vi "UART Clear Buffer.vi"(5 "Error In":errorcluster, 8 "VISA Resource In":refnum<visa-resource-name>="COM1") -> (0 "Error Out":errorcluster, 3 "VISA Resource Out":refnum<visa-resource-name>)   [LabVIEW 2015]
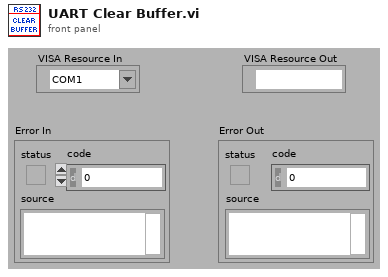
[diagram p1: front panel]
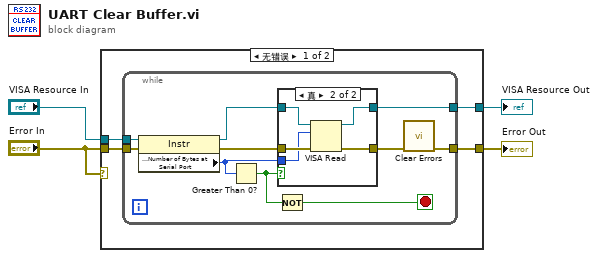
[diagram p0: block diagram]
diagram:
  n1 = case shown="无错误" "Error In" {
    tunnel: "VISA Resource In" -> [w8 w27]
    tunnel: "Error In" -> [w7 w26]
    tunnel: [w6 w26] -> w3
    tunnel: [w5 w27] -> w2
    frame No Error {
      n2 = while {
        tunnel: w8 -> [w18]
        tunnel: w7 -> [w17]
        tunnel: [w11] -> w6
        tunnel: [w16] -> w5
        stop <- w9 stop-if-true
        n3 = property class="Instr"(reference=w18, error in=w17) -> (reference out=w15:refnum<visa-resource-name>, error out=w14:errorcluster, "Serial Settings:Number of Bytes at Serial Port"=w13:u32)
        n4 = Greater Than 0?(x=w13) -> (x > 0?=w10:bool)
        n5 = Not(x=w10) -> (.not. x?=w9:bool)
        n6 = case shown="真" w10 {
          tunnel: w15 -> [w19 w25]
          tunnel: w14 -> [w20 w24]
          tunnel: w13 -> [_ w23]
          tunnel: [w20 w22] -> w12
          tunnel: [w19 w21] -> w16
          frame False {
          }
          frame True {
            n7 = VISA Read(VISA resource name=w25, byte count=w23, error in (no error)=w24) -> (VISA resource name out=w21:refnum<visa-resource-name>, error out=w22:errorcluster)  [unwired: 2 out]
          }
        }
        n8 = call <vilib>:"Clear Errors.vi"("error in (no error)"=w12) -> ("error out"=w11:errorcluster)  [unwired: 5 in, 1 out]
      }
    }
    frame Error {
    }
  }
  "VISA Resource Out" <- w2
  "Error Out" <- w3
